vi "affichage_registre_decalage.vi"() -> ()   [LabVIEW 2013]
panel:
  in  "Booléen":bool
  out "t":i32
  out "t-3":i32
  out "t- 2":i32
  out "t-1":i32
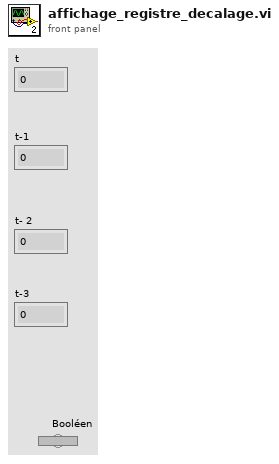
[diagram p1: front panel]
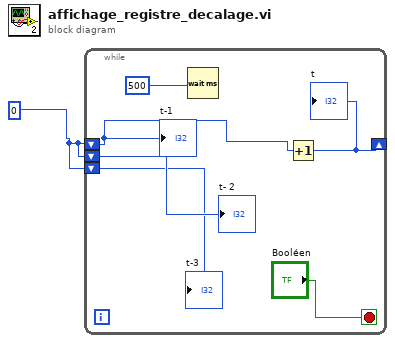
[diagram p0: block diagram]
diagram:
  w1 = 0
  n1 = while {
    shift-right: [w3] -> _
    shift-left: w1 -> [w4]
    shift-left: w1 -> [w6]
    shift-left: w1 -> [w5]
    stop <- "Booléen" stop-if-true
    n2 = Wait (ms)(milliseconds to wait=500) -> ()  [unwired: 1 out]
    n3 = Increment(x=w4) -> (x+1=w3:i32)
    "t" <- w3
    "t-1" <- w4
    "t- 2" <- w6
    "t-3" <- w5
  }
